vi "TwRegisterUserDataWrite.vi"(0 "location":string, 1 "nbrElements":i32, 2 "elementDescription":u8[](array[numeric]), 3 "compressionLevel":i32, 4 "error in (no error)":errorcluster) -> (5 "error out":errorcluster)   [LabVIEW 2009]
uses:
  TofDaqDll.dll
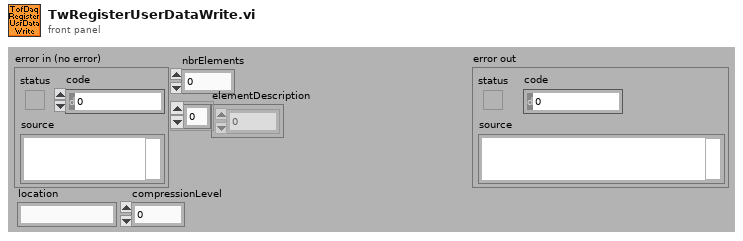
[diagram p1: front panel]
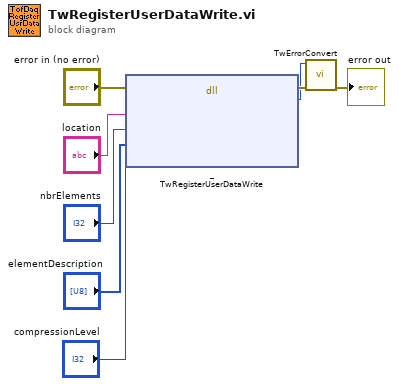
[diagram p0: block diagram]
diagram:
  n1 = dll-call lib="C:/src/TofDaq/APIandWrappers/LabView/TofDaqDll/TofDaqDll.dll" fn="_TwRegisterUserDataWrite"(error in="error in (no error)", "location"="location", "nbrElements"="nbrElements", "elementDescription"="elementDescription", "compressionLevel"="compressionLevel") -> (error out=w7:errorcluster, "TwRetVal"=w5:i32)  [unwired: 6 in, 1 out]
  n2 = call "TwErrorConvert.vi"("error in (no error)"=w7, "error code"=w5) -> ("error out"=→"error out":errorcluster)  [unwired: 9 out]
